vi "Sequence State Machine.vi"(8 "error in (no error)":errorcluster, 10 "Current time":timestamp, 11 "Output Sequencer in":refnum<class "Output Sequencer.lvclass">) -> (0 "error out":errorcluster, 3 "Output Sequencer out":refnum<class "Output Sequencer.lvclass">)   [LabVIEW 2020, in "Output Sequencer.lvlib" / "Output Sequencer.lvclass"]
uses:
  Output Sequencer.lvclass
  Output Sequencer.lvclass/Output Sequencer.ctl
  Types/Sequencer State.ctl
  <vilib>/FlexLogger/SDK/PluginSDK.lvlibp
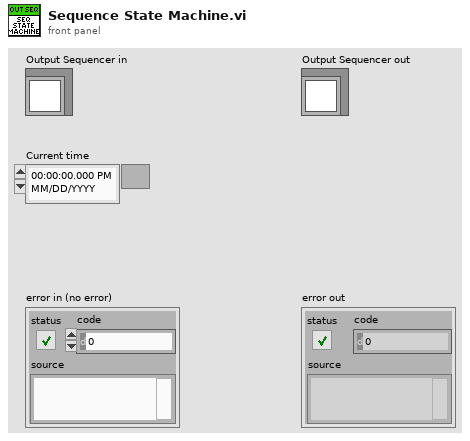
[diagram p1: front panel]
types:
  T1 = typedef "Output Sequencer.lvlib/Output Sequencer.lvclass/Sequencer State.ctl" = enum16{"Error", "Initialize", "Prepare channels", "Wait for test", "Wait for %.1f sec", "Wait for trigger", "Stop condition", "Wait for resume", "Running", "Paused", "No valid step", "Stopped"}
  T2 = typedef "Output Sequencer.lvlib/Output Sequencer.lvclass/Expression Data.ctl" = cluster{"Empty?":bool, "Expression":refnum<class "mupExpr.lvclass">, "Variable Names":string[]}
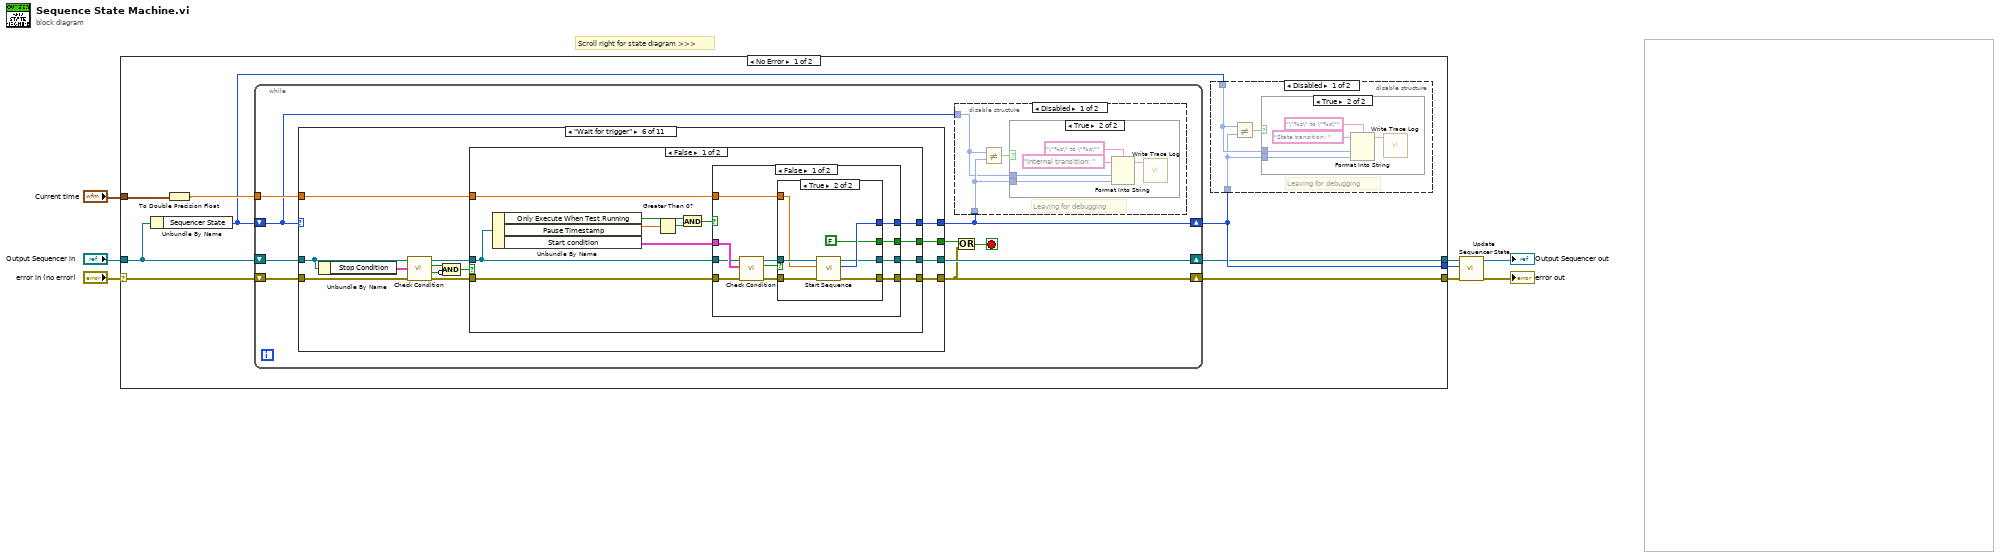
[diagram p0: block diagram]
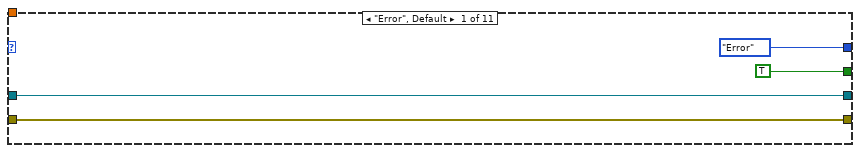
[diagram p6: hidden frame]
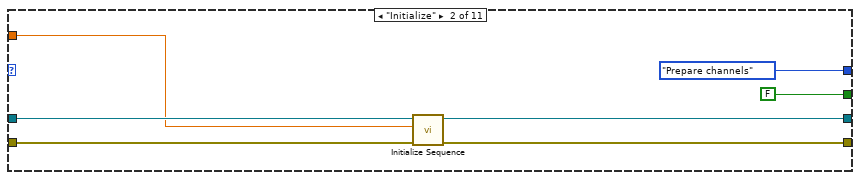
[diagram p7: hidden frame]
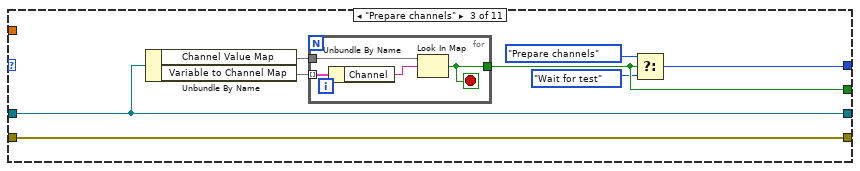
[diagram p8: hidden frame]
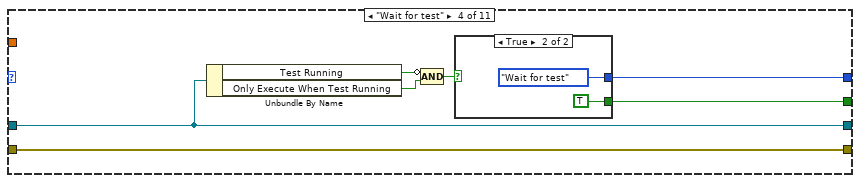
[diagram p9: hidden frame]
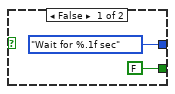
[diagram p10: hidden frame]
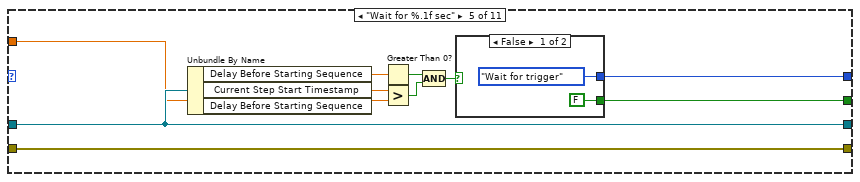
[diagram p11: hidden frame]
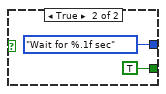
[diagram p12: hidden frame]
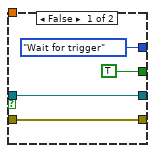
[diagram p13: hidden frame]
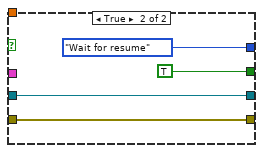
[diagram p14: hidden frame]
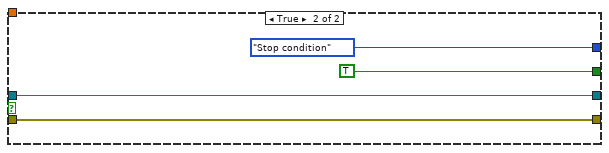
[diagram p15: hidden frame]
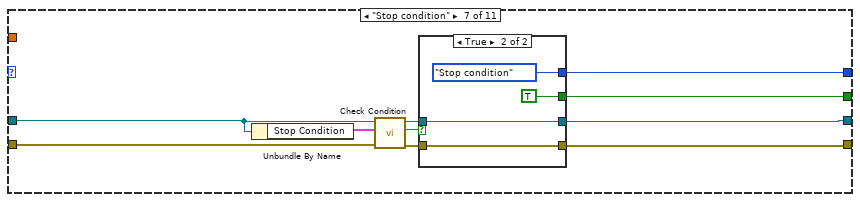
[diagram p16: hidden frame]
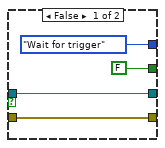
[diagram p17: hidden frame]
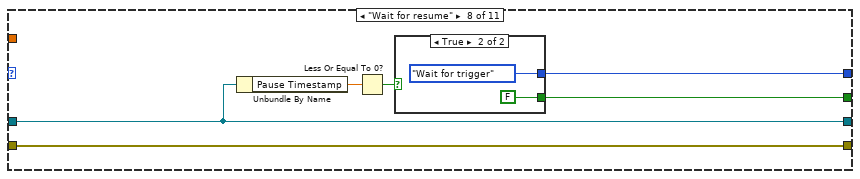
[diagram p18: hidden frame]
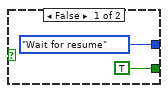
[diagram p19: hidden frame]
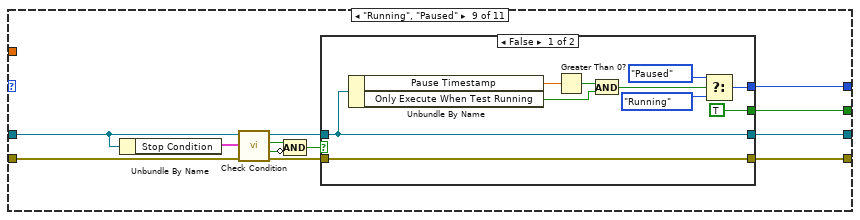
[diagram p20: hidden frame]
diagram:
  # "Scroll right for state diagram >>>"
  n1 = case shown="No Error" "error in (no error)" {
    selector: "error in (no error)" -> [w9 w255]
    tunnel: "Output Sequencer in" -> [w16 w256]
    tunnel: "Current time" -> [w15 _]
    tunnel: [w12 w255] -> w6
    tunnel: [w11 _] -> w5
    tunnel: [w10 w256] -> w3
    frame No Error {
      n2 = Unbundle By Name(w16) -> ("Sequencer State"=w13:T1)
      n3 = To Double Precision Float(number=w15) -> (double precision float=w14:dbl)
      n4 = while {
        shift-right: [w30] -> w11
        shift-left: w13 -> [w28]
        shift-right: [w32] -> w10
        shift-left: w16 -> [w33]
        tunnel: w14 -> [w31]
        shift-right: [w26] -> w12
        shift-left: w9 -> [w29]
        stop <- w25 stop-if-true
        n5 = case shown="\"Wait for trigger\"" w28 {
          tunnel: w33 -> [w43 w50 w60 w71 w85 w95 w153 w164 w184 w204 w250]
          tunnel: [Sequencer_State."Error" ("State.Sequencer State") Sequencer_State."Prepare channels" ("State.Sequencer State") w59 w70 w84 w102 w150 w166 w180 w205 w248] -> w30
          tunnel: [w43 w51 w60 w71 w85 w99 w148 w164 w181 w207 w250] -> w32
          tunnel: [TRUE FALSE ("Boolean") w55 w69 w77 w101 w149 w165 w179 w202 w247] -> w27
          tunnel: w31 -> [_ w49 _ _ w81 w100 _ _ _ w201 _]
          tunnel: w29 -> [w42 w47 w58 w65 w76 w92 w147 w163 w175 w208 w239]
          tunnel: [w42 w46 w58 w65 w76 w90 w145 w163 w173 w206 w239] -> w26
          frame "Error", Default {
          }
          frame "Initialize" {
            n6 = call "Initialize Sequence.vi"("error in (no error)"=w47, "Current Time"=w49, "Output Sequencer in"=w50) -> ("error out"=w46:errorcluster, "Output Sequencer out"=w51:refnum<class "Output Sequencer.lvclass">)  [unwired: 7 in]
          }
          frame "Prepare channels" {
            n7 = Unbundle By Name(w60) -> ("Channel Value Map"=w56:map{string, dbl}, "Variable to Channel Map"=w57:map{string, string})
            n8 = for {
              tunnel: w57 -> [w64] mode=indexing
              tunnel: w56 -> [w62]
              tunnel: [w61] -> w55
              stop <- w61 stop-if-true
              n9 = Unbundle By Name(w64) -> ("Channel"=w63:string)
              n10 = Look In Map(map=w62, key=w63) -> (key not found?=w61:bool)  [unwired: 1 in, 1 out]
            }
            n11 = Select(t=Sequencer_State."Prepare channels" ("State.Sequencer State"), s=w55, f=Sequencer_State."Wait for test" ("State.Sequencer State")) -> (s? t:f=w59:T1)
          }
          frame "Wait for test" {
            n12 = Unbundle By Name(w71) -> ("Test Running"=w68:bool, "Only Execute When Test Running"=w67:bool)
            n13 = Compound Arithmetic op=AND(invert w68, w67) -> (w66:bool)
            n14 = case shown="True" w66 {
              tunnel: [Sequencer_State."Wait for %.1f sec" ("State.Sequencer State") Sequencer_State."Wait for test" ("State.Sequencer State")] -> w70
              tunnel: [FALSE TRUE] -> w69
              frame False {
              }
              frame True {
              }
            }
          }
          frame "Wait for %.1f sec" {
            n15 = Unbundle By Name(w85) -> ("Delay Before Starting Sequence"=w83:dbl, "Current Step Start Timestamp"=w80:dbl)  [unwired: 1 out]
            n16 = Greater Than 0?(x=w83) -> (x > 0?=w82:bool)
            n17 = Greater?(x=w80, y=w81) -> (0:w79:bool)
            n18 = Compound Arithmetic op=AND(w82, w79) -> (w78:bool)
            n19 = case shown="False" w78 {
              tunnel: [Sequencer_State."Wait for trigger" ("State.Sequencer State") Sequencer_State."Wait for %.1f sec" ("State.Sequencer State")] -> w84
              tunnel: [FALSE TRUE] -> w77
              frame False {
              }
              frame True {
              }
            }
          }
          frame "Wait for trigger" {
            n20 = Unbundle By Name(w95) -> ("Stop Condition"=w98:T2)
            n21 = call "Check Condition.vi"("error in (no error)"=w92, "Expression Data"=w98, "Output Sequencer in"=w95) -> ("error out"=w91:errorcluster, "Condition empty"=w96:bool, "Check passed"=w97:bool, "Output Sequencer out"=w93:refnum<class "Output Sequencer.lvclass">)  [unwired: 5 in]
            n22 = Compound Arithmetic op=AND(w97, invert w96) -> (w94:bool)
            n23 = case shown="False" w94 {
              tunnel: [w114 Sequencer_State."Stop condition" ("State.Sequencer State")] -> w102
              tunnel: [w113 TRUE] -> w101
              tunnel: w100 -> [w112 _]
              tunnel: [w111 w143] -> w99
              tunnel: w93 -> [w106 w143]
              tunnel: w91 -> [w105 w141]
              tunnel: [w104 w141] -> w90
              frame False {
                n24 = Unbundle By Name(w106) -> ("Only Execute When Test Running"=w108:bool, "Pause Timestamp"=w110:dbl, "Start condition"=w103:T2)
                n25 = Greater Than 0?(x=w110) -> (x > 0?=w109:bool)
                n26 = And(x=w108, y=w109) -> (x .and. y?=w107:bool)
                n27 = case shown="False" w107 {
                  tunnel: [w125 Sequencer_State."Wait for resume" ("State.Sequencer State")] -> w114
                  tunnel: [w124 TRUE] -> w113
                  tunnel: w103 -> [w123 _]
                  tunnel: w112 -> [w120 _]
                  tunnel: [w119 w138] -> w111
                  tunnel: w106 -> [w118 w138]
                  tunnel: w105 -> [w117 w137]
                  tunnel: [w115 w137] -> w104
                  frame False {
                    n28 = call "Check Condition.vi"("error in (no error)"=w117, "Expression Data"=w123, "Output Sequencer in"=w118) -> ("error out"=w116:errorcluster, "Check passed"=w121:bool, "Output Sequencer out"=w122:refnum<class "Output Sequencer.lvclass">)  [unwired: 5 in, 1 out]
                    n29 = case shown="True" w121 {
                      tunnel: [Sequencer_State."Wait for trigger" ("State.Sequencer State") w136] -> w125
                      tunnel: [TRUE FALSE] -> w124
                      tunnel: w122 -> [w129 w134]
                      tunnel: w120 -> [_ w132]
                      tunnel: [w129 w133] -> w119
                      tunnel: w116 -> [w126 w131]
                      tunnel: [w126 w130] -> w115
                      frame False {
                      }
                      frame True {
                        n30 = call "Start Sequence.vi"("error in (no error)"=w131, "Current Time"=w132, "Output Sequencer in"=w134) -> ("error out"=w130:errorcluster, "Sequencer State"=w136:T1, "Output Sequencer out"=w133:refnum<class "Output Sequencer.lvclass">)  [unwired: 6 in]
                      }
                    }
                  }
                  frame True {
                  }
                }
              }
              frame True {
              }
            }
          }
          frame "Stop condition" {
            n31 = Unbundle By Name(w153) -> ("Stop Condition"=w154:T2)
            n32 = call "Check Condition.vi"("error in (no error)"=w147, "Expression Data"=w154, "Output Sequencer in"=w153) -> ("error out"=w146:errorcluster, "Check passed"=w152:bool, "Output Sequencer out"=w151:refnum<class "Output Sequencer.lvclass">)  [unwired: 5 in, 1 out]
            n33 = case shown="True" w152 {
              tunnel: w151 -> [w158 w160]
              tunnel: [w158 w160] -> w148
              tunnel: [Sequencer_State."Wait for trigger" ("Sequencer State") Sequencer_State."Stop condition" ("Sequencer State")] -> w150
              tunnel: [FALSE TRUE] -> w149
              tunnel: w146 -> [w155 w159]
              tunnel: [w155 w159] -> w145
              frame False {
              }
              frame True {
              }
            }
          }
          frame "Wait for resume" {
            n34 = Unbundle By Name(w164) -> ("Pause Timestamp"=w168:dbl)
            n35 = Less Or Equal To 0?(x=w168) -> (x <= 0?=w167:bool)
            n36 = case shown="True" w167 {
              tunnel: [Sequencer_State."Wait for resume" ("State.Sequencer State") Sequencer_State."Wait for trigger" ("State.Sequencer State")] -> w166
              tunnel: [TRUE ("Boolean") FALSE ("Boolean")] -> w165
              frame False {
              }
              frame True {
              }
            }
          }
          frame "Running", "Paused" {
            n37 = Unbundle By Name(w184) -> ("Stop Condition"=w178:T2)
            n38 = call "Check Condition.vi"("error in (no error)"=w175, "Expression Data"=w178, "Output Sequencer in"=w184) -> ("error out"=w174:errorcluster, "Condition empty"=w176:bool, "Check passed"=w177:bool, "Output Sequencer out"=w182:refnum<class "Output Sequencer.lvclass">)  [unwired: 5 in]
            n39 = Compound Arithmetic op=AND(w177, invert w176) -> (w183:bool)
            n40 = case shown="False" w183 {
              tunnel: w182 -> [w194 w200]
              tunnel: [w194 w199] -> w181
              tunnel: [w193 w198] -> w180
              tunnel: [TRUE ("Boolean") FALSE ("Boolean")] -> w179
              tunnel: w174 -> [w185 w196]
              tunnel: [w185 w195] -> w173
              frame False {
                n41 = Unbundle By Name(w194) -> ("Pause Timestamp"=w191:dbl, "Only Execute When Test Running"=w188:bool)
                n42 = Greater Than 0?(x=w191) -> (x > 0?=w189:bool)
                n43 = And(x=w189, y=w188) -> (x .and. y?=w187:bool)
                n44 = Select(t=Sequencer_State."Paused" ("State.Sequencer State"), s=w187, f=Sequencer_State."Running") -> (s? t:f=w193:T1)
              }
              frame True {
                n45 = call "Stop Sequence.vi"("error in (no error)"=w196, "Output Sequencer in"=w200) -> ("error out"=w195:errorcluster, "Sequencer State"=w198:T1, "Output Sequencer out"=w199:refnum<class "Output Sequencer.lvclass">)  [unwired: 7 in]
              }
            }
          }
          frame "No valid step" {
            n46 = Unbundle By Name(w204) -> ("Current Step"=w203:i32)
            n47 = call "Find Valid Step.vi"("error in (no error)"=w208, "Starting Step"=w203, "Output Sequencer in"=w204) -> ("error out"=w210:errorcluster, "Next Cycle?"=w213:bool, "Next Step"=w211:i32, "Output Sequencer out"=w212:refnum<class "Output Sequencer.lvclass">, "Valid Step Found"=w209:bool)  [unwired: 4 in]
            n48 = case shown="True" w209 {
              tunnel: [w216 w238] -> w206
              tunnel: [w217 w237] -> w207
              tunnel: w213 -> [_ w232]
              tunnel: w212 -> [w217 w222]
              tunnel: w211 -> [_ w228]
              tunnel: w210 -> [w216 w223]
              tunnel: [Sequencer_State."No valid step" ("Sequencer State") w233] -> w205
              tunnel: [TRUE ("Max iterations reached?") w229] -> w202
              tunnel: w201 -> [_ w218]
              frame False {
              }
              frame True {
                n49 = Unbundle By Name(w222) -> ("Pause Timestamp"=w226:dbl, "Total Iterations"=w231:i32)
                n50 = Greater Than 0?(x=w226) -> (x > 0?=w227:bool)
                n51 = Increment(x=w231) -> (x+1=w235:i32)
                n52 = Select(t=w235, s=w232, f=w231) -> (s? t:f=w234:i32)
                n53 = Select(t=w218, s=w227, f=0.0) -> (s? t:f=w224:dbl)
                n54 = call "Get Current Step Duration.vi"("error in (no error)"=w223, "Output Sequencer in"=w222) -> ("error out"=w220:errorcluster, "Duration"=w219:dbl, "Output Sequencer out"=w221:refnum<class "Output Sequencer.lvclass">)  [unwired: 7 in]
                n55 = Bundle By Name(cluster=w221, "Pause Timestamp"=w224, "Current Step Start Timestamp"=w218, "Total Iterations"=w234, "Sequencer State"=Sequencer_State."Running" ("State.Sequencer State"), "Current Step"=w228, "Time Remaining"=w219) -> (w236:refnum<class "Output Sequencer.lvclass">)
                n56 = call "Check Max Cycles.vi"("error in (no error)"=w220, "Output Sequencer in"=w236) -> ("error out"=w238:errorcluster, "Max iterations reached?"=w229:bool, "Output Sequencer out"=w237:refnum<class "Output Sequencer.lvclass">, "Sequencer State"=w233:T1)  [unwired: 6 in]
              }
            }
          }
          frame "Stopped" {
            n57 = Unbundle By Name(w250) -> ("Start condition"=w243:string, "Enable re-triggering"=w242:bool, "Test Running"=w246:bool, "Only Execute When Test Running"=w245:bool)
            n58 = Empty String/Path?(string/path=w243) -> (empty?=w244:bool)
            n59 = Compound Arithmetic op=AND(invert w244, w242) -> (w241:bool)
            n60 = Compound Arithmetic op=AND(invert w246, w245) -> (w240:bool)
            n61 = Compound Arithmetic op=OR(w241, w240) -> (w249:bool)
            n62 = case shown="True" w249 {
              tunnel: [Sequencer_State."Stopped" ("State.Sequencer State") Sequencer_State."Wait for test" ("State.Sequencer State")] -> w248
              tunnel: [TRUE ("Boolean") FALSE ("Boolean")] -> w247
              frame False {
              }
              frame True {
              }
            }
          }
        }
        n63 = disable-structure shown="Disabled" {
          disable-tunnel: w30 -> [w36 _]
          disable-tunnel: w28 -> [w34 _]
          frame Disabled {
            # "Leaving for debugging"
            n64 = Not Equal?(x=w34, y=w36) -> (x != y?=w35:bool)
            n65 = case shown="True" w35 {
              tunnel: w34 -> [_ w38]
              tunnel: w36 -> [_ w37]
              frame False {
              }
              frame True {
                n66 = Format Into String(format string="\"%s\" to \"%s\"", initial string="Internal transition: ", w38, w37) -> (resulting string=w41:string)  [unwired: 1 in, 1 out]
                n67 = call <vilib>:"Write Trace Log.vi"("Message"=w41) -> ()  [unwired: 10 in, 1 out]
              }
            }
          }
          frame Enabled {
          }
        }
        n68 = Or(x=w27, y=w26) -> (x .or. y?=w25:bool)
      }
      n69 = disable-structure shown="Disabled" {
        disable-tunnel: w13 -> [w18 _]
        disable-tunnel: w11 -> [w17 _]
        frame Disabled {
          # "Leaving for debugging"
          n70 = Not Equal?(x=w18, y=w17) -> (x != y?=w19:bool)
          n71 = case shown="True" w19 {
            tunnel: w18 -> [_ w21]
            tunnel: w17 -> [_ w20]
            frame False {
            }
            frame True {
              n72 = Format Into String(format string="\"%s\" to \"%s\"", initial string="State transition: ", w21, w20) -> (resulting string=w24:string)  [unwired: 1 in, 1 out]
              n73 = call <vilib>:"Write Trace Log.vi"("Message"=w24) -> ()  [unwired: 10 in, 1 out]
            }
          }
        }
        frame Enabled {
        }
      }
    }
    frame Error {
    }
  }
  n74 = call "Update Sequencer State.vi"("error in (no error)"=w6, "Sequencer State"=w5, "Output Sequencer in"=w3) -> ("error out"=→"error out":errorcluster, "Output Sequencer out"=→"Output Sequencer out":refnum<class "Output Sequencer.lvclass">)  [unwired: 7 in]
